vi "Goto_A.vi"(0 "reference":refnum<visa-resource-name>, 7 "Axis Number":u8(ring)=1 items=["", "1", "2", "3", "4"], 9 "Direction":bool, 11 "Pulse Number":i32=100 min=1 max=500000) -> (4 "reference dup":refnum<visa-resource-name>, 8 "OK Done":bool, 15 "error OUT":errorcluster)   [LabVIEW 2011]
panel:
  # "Port Number 0=COM1"
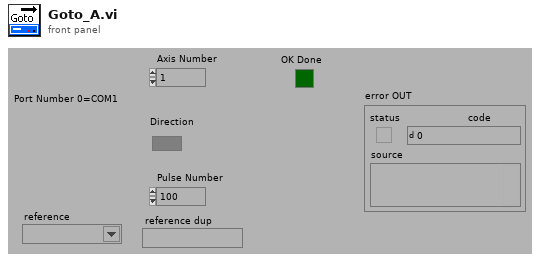
[diagram p1: front panel]
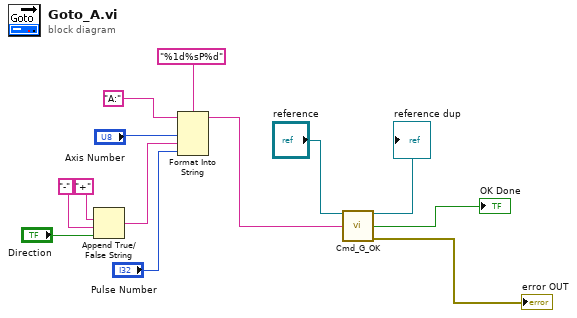
[diagram p0: block diagram]
diagram:
  n1 = Append True/False String(1:"Direction", 2:"-", 3:"+") -> (0:w6:string)  [unwired: 1 in]
  n2 = Format Into String(format string="%1d%sP%d", initial string="A:", "Axis Number", w6, "Pulse Number") -> (resulting string=w5:string)  [unwired: 1 in, 1 out]
  n3 = call "Cmd_G_OK.vi"("reference"="reference", "Command String"=w5) -> ("reference dup"=→"reference dup":refnum<visa-resource-name>, "OK Done"=→"OK Done":bool, "error OUT"=→"error OUT":errorcluster)  [unwired: 11 in]
